vi "Step Association Update.vi"(8 "error in (no error)":errorcluster, 10 "Step Association Record (empty)":T2, 11 "Connection Refnum":T1) -> (0 "error out":errorcluster, 3 "Connection Refnum":T1)   [LabVIEW 2011]
uses:
  Step Association Record.ctl
  SI.LIB/ODBC/SQL Controls/Connection Refnum.ctl
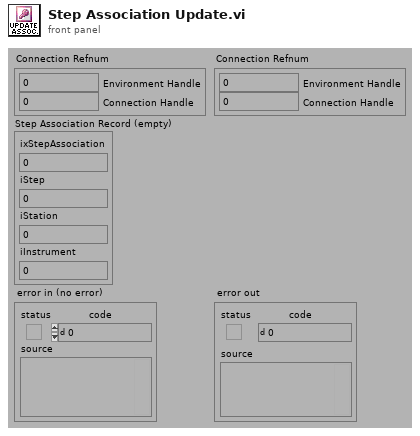
[diagram p1: front panel]
types:
  T1 = typedef "Connection Refnum.ctl" = cluster{"Environment Handle":i32, "Connection Handle":i32}
  T2 = typedef "Step Association Record.ctl" = cluster{"ixStepAssociation":i32, "iStep":i32, "iStation":i32, "iInstrument":i32}
  T3 = typedef "Statement Refnum.ctl" = cluster{"Statement Handle":i32, "Parameter Number":u16}
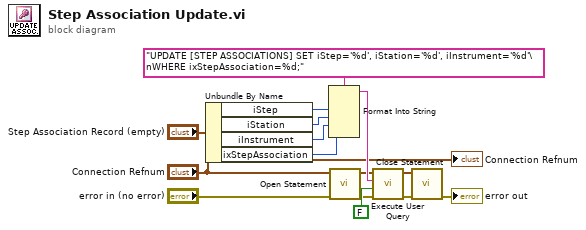
[diagram p0: block diagram]
diagram:
  n1 = Unbundle By Name("Step Association Record (empty)") -> ("iStep"=w1:i32, "iStation"=w6:i32, "iInstrument"=w5:i32, "ixStepAssociation"=w7:i32)
  n2 = Format Into String(format string="UPDATE [STEP ASSOCIATIONS] SET iStep='%d', iStation='%d', iInstrument='%d'\nWHERE ixStepAssociation=%d;" ("User Query"), w1, w6, w5, w7) -> (resulting string=w10:string)  [unwired: 2 in, 1 out]
  n3 = call "Open Statement.vi"("error in (no error)"="error in (no error)", "Connection Refnum"="Connection Refnum") -> ("error out"=w9:errorcluster, "Statement Refnum"=w8:T3)  [unwired: 4 out]
  n4 = call "Execute User Query.vi"("error in (no error)"=w9, "Return Data? (f)"=FALSE, "User Query"=w10, "Statement Refnum"=w8) -> ("error out"=w13:errorcluster, "Statement Refnum"=w12:T3)  [unwired: 2 out]
  n5 = call "Close Statement.vi"("error in (no error)"=w13, "Statement Refnum"=w12) -> ("error out"=→"error out":errorcluster)  [unwired: 5 out]
  "Connection Refnum" <- "Connection Refnum"
